vi "testExample 1.vi"(8 "error in (no error)":errorcluster, 11 "TestCase in":refnum<class "JKI VI Tester Add Test.lvclass">) -> (0 "error out":errorcluster, 3 "TestCase out":refnum<class "JKI VI Tester Add Test.lvclass">)   [LabVIEW 2018, in "JKI VI Tester Add TEst.lvclass"]
uses:
  JKI VI Tester Add Test.lvclass
  <vilib>/addons/_JKI Toolkits/VI Tester/TestCase.llb/TestCase.lvclass
  C:/Program Files (x86)/National Instruments/LabVIEW 2018/vi.lib/addons/_JKI Toolkits/VI Tester/TestCase.llb/TestCase.lvclass
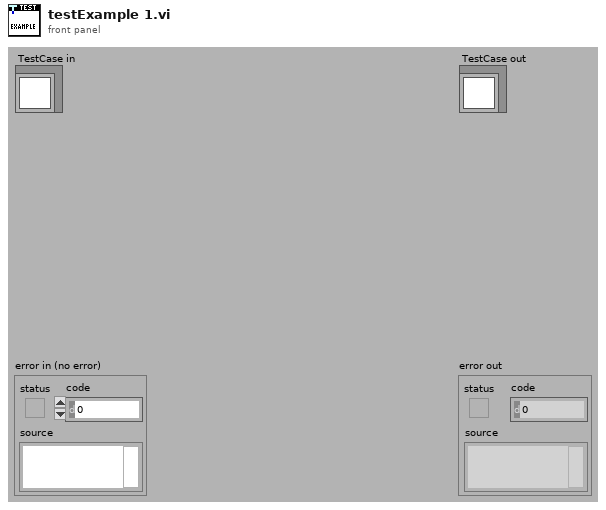
[diagram p1: front panel]
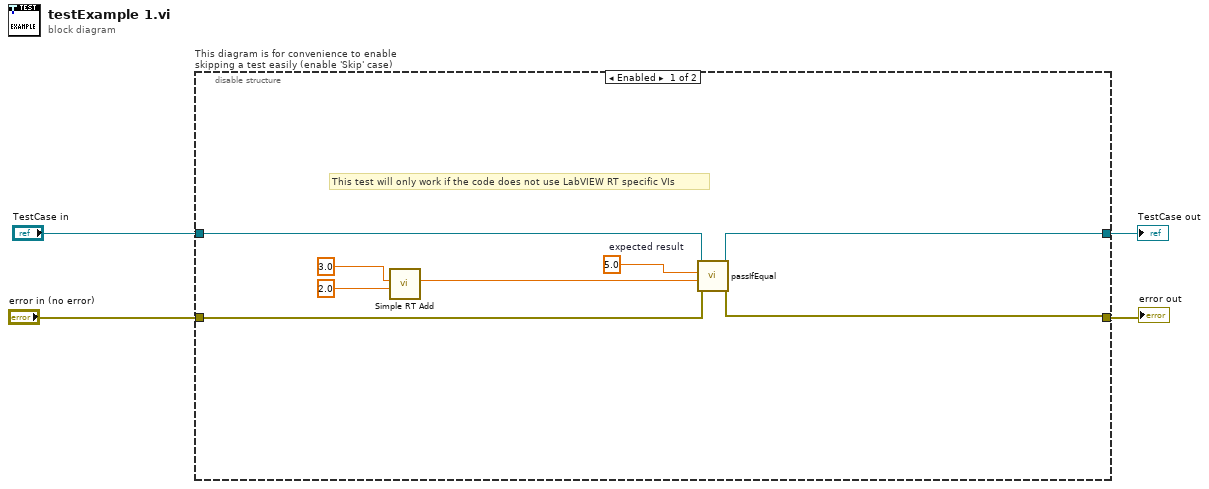
[diagram p0: block diagram]
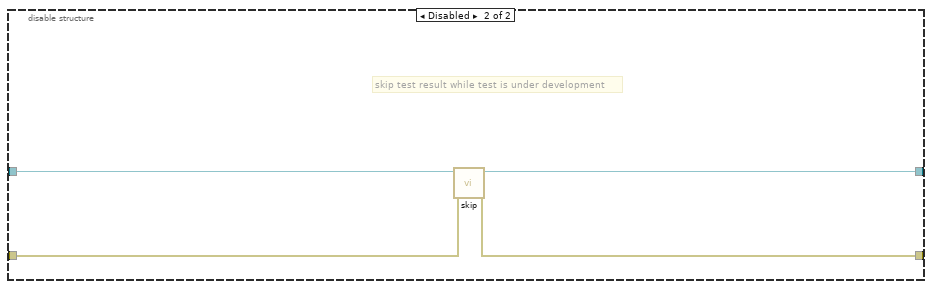
[diagram p2: hidden frame]
diagram:
  n1 = disable-structure "This diagram is for convenience to enable skipping a test easily (enable 'Skip' case)" shown="Enabled" {
    disable-tunnel: "TestCase in" -> [w11 w16]
    disable-tunnel: [w10 w14] -> w1
    disable-tunnel: [w9 w15] -> w3
    disable-tunnel: "error in (no error)" -> [w8 w13]
    frame Enabled {
      w12 = 5.0  # expected result
      # "This test will only work if the code does not use LabVIEW RT specific VIs"
      n2 = call "Simple RT Add.vi"("y"=2.0, "x"=3.0) -> ("x+y"=w5:dbl)  [unwired: 9 in]
      n3 = call-dynamic "passIfEqual.vi"("error in (no error)"=w8, "y"=w5, "x"=w12, "TestCase in"=w11) -> ("error out"=w9:errorcluster, "TestCase out"=w10:refnum<class "JKI VI Tester Add Test.lvclass">)  [unwired: 6 in]
    }
    frame Disabled {
      # "skip test result while test is under development"
      n4 = call <vilib>:"skip.vi"("error in (no error)"=w13, "TestCase in"=w16) -> ("error out"=w15:errorcluster, "TestCase out"=w14:refnum<class "JKI VI Tester Add Test.lvclass">)  [unwired: 8 in]
    }
  }
  "error out" <- w3
  "TestCase out" <- w1
